vi "PWMcontroller.vi"(3 "Duty Cycle [0-100%]":dbl, 4 "Period [ms]":dbl, 5 "Count in":u32) -> (1 "State":bool, 2 "Count out":u32)   [LabVIEW 2020]
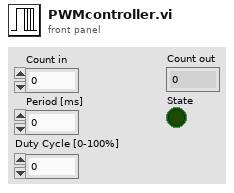
[diagram p1: front panel]
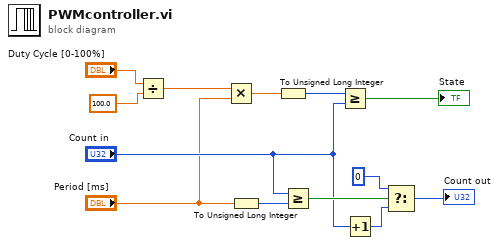
[diagram p0: block diagram]
diagram:
  n1 = Divide(x="Duty Cycle [0-100%]", y=100.0) -> (x/y=w2:dbl)
  n2 = Multiply(x=w2, y="Period [ms]") -> (x*y=w13:dbl)
  n3 = To Unsigned Long Integer(number="Period [ms]") -> (unsigned 32bit integer=w10:u32)
  n4 = To Unsigned Long Integer(number=w13) -> (unsigned 32bit integer=w4:u32)
  n5 = Greater Or Equal?(x="Count in", y=w10) -> (x >= y?=w9:bool)
  n6 = Greater Or Equal?(x=w4, y="Count in") -> (x >= y?=→"State":bool)
  n7 = Increment(x="Count in") -> (x+1=w8:u32)
  n8 = Select(t=u32 0, s=w9, f=w8) -> (s? t:f=→"Count out":u32)
